vi "SetGroupProperty.vi"(7 "LabVIEW Web Service Request":refnum<class "Web Request.lvclass">) -> ()   [LabVIEW 2018]
uses:
  <vilib>/wsapi/Web Request.lvclass
  subvis/Group Properties.ctl
  CAEN globals.vi
panel:
  in  "error in (no error)":errorcluster
  # "Use the Web Service Request input terminal to call the VIs on the Web Services palette. Do not remove it from the connector pane unless you don't need access to the palette."
  # "Each additional control wired to the connector pane will be available as an input in the URL. To include an indicator in terminal-mode output (the default setting), it must also be wired to the connector pane."
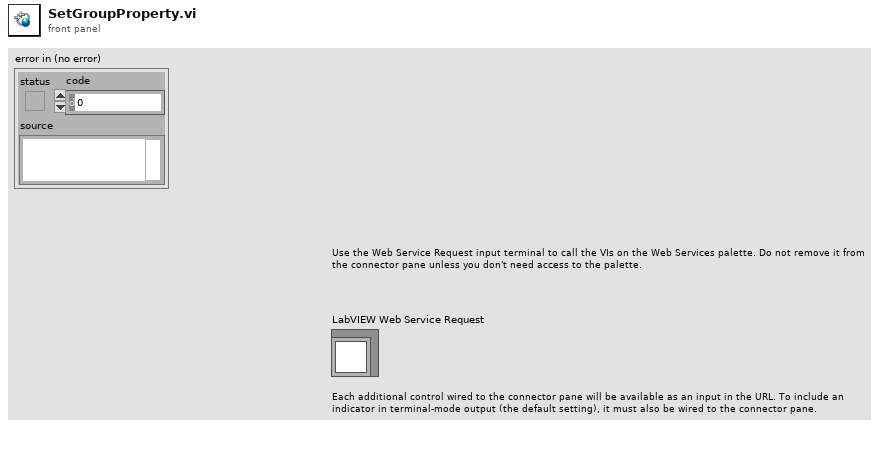
[diagram p1: front panel]
types:
  T1 = typedef "Group Properties.ctl" = enum16{"Enable", "Vset", "Imax", "Vswmax", "Trip Time"}
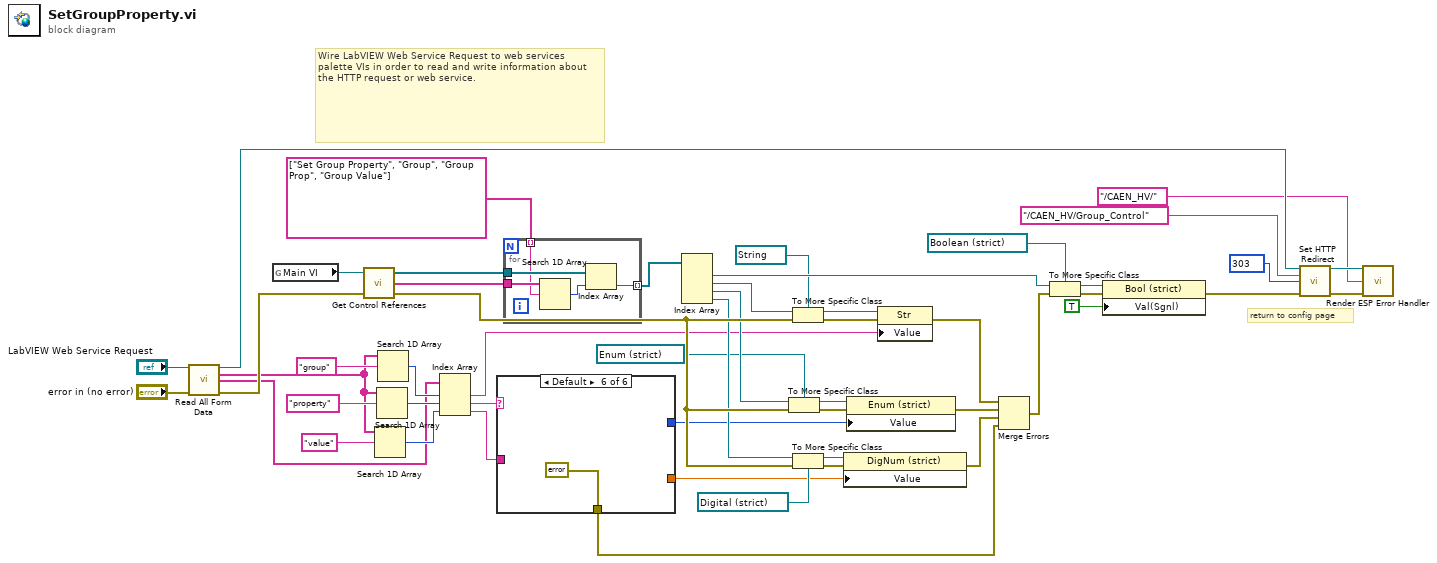
[diagram p0: block diagram]
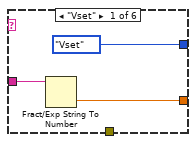
[diagram p2: hidden frame]
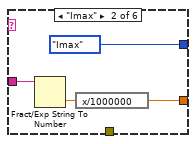
[diagram p3: hidden frame]
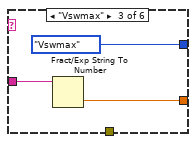
[diagram p4: hidden frame]
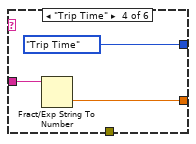
[diagram p5: hidden frame]
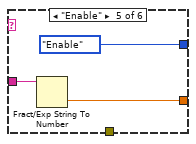
[diagram p6: hidden frame]
diagram:
  w46 = 303 items=["100"=100, "101"=101, "200"=200, "201"=201, "202"=202, "203"=203, "204"=204, "205"=205, "206"=206, "300"=300, "301"=301, "302"=302, "303"=303, "304"=304, "305"=305, "306"=306, "307"=307, "400"=400, "401"=401, "402"=402, "403"=403, "404"=404, "405"=405, "406"=406, "407"=407, "408"=408, "409"=409, "410"=410, "411"=411, "412"=412, "413"=413, "414"=414, "415"=415, "416"=416, "417"=417, "500"=500, "501"=501, "502"=502, "503"=503, "504"=504, "505"=505] ("response code (307)")
  # "return to config page"
  # "Wire LabVIEW Web Service Request to web services palette VIs in order to read and write information about the HTTP request or web service."
  n1 = call <vilib>:"Read All Form Data.vi"("LabVIEW Web Service Request"="LabVIEW Web Service Request", "error in (no error)"="error in (no error)") -> ("LabVIEW Web Service Request out"=w22:refnum<class "Web Request.lvclass">, "Key"=w14:string[], "Value"=w12:string[], "error out"=w23:errorcluster)  [unwired: 9 in, 1 out]
  n2 = global read "CAEN globals.vi" "Main VI"() -> (w51:refnum<vi>)
  n3 = call "Get Control References.vi"("error in"=w23, "This vi"=w51) -> ("error out"=w25:errorcluster, "Control Names"=w50:string[], "Controls[]"=w49:refnum<vi>[])  [unwired: 1 in]
  n4 = Search 1D Array(1D array=w14, element="value") -> (index of element=w13:i32)  [unwired: 1 in]
  n5 = Search 1D Array(1D array=w14, element="property") -> (index of element=w41:i32)  [unwired: 1 in]
  n6 = Search 1D Array(1D array=w14, element="group") -> (index of element=w42:i32)  [unwired: 1 in]
  n7 = Index Array(array=w12, index #1=w42, index #2=w41, index #3=w13) -> (element #1=w8:string, element #2=w5:string, element #3=w3:string)
  n8 = case shown="Default" w5 {
    tunnel: [Group_Properties."Vset" ("Value") Group_Properties."Imax" ("Value") Group_Properties."Vswmax" ("Value") Group_Properties."Trip Time" ("Value") Group_Properties."Enable" ("Value") _] -> w4
    tunnel: w3 -> [w53 w56 w60 w63 w66 _]
    tunnel: [w52 w55 w59 w62 w65 _] -> w2
    tunnel: [_ _ _ _ _ errorcluster {"status"=TRUE, "code"=0, "source"="Unrecognised group property"} ("error out")] -> w1
    frame "Vset" {
      n9 = Fract/Exp String To Number(string=w53) -> (number=w52:dbl)  [unwired: 3 in, 1 out]
    }
    frame "Imax" {
      n10 = Fract/Exp String To Number(string=w56) -> (number=w57:dbl)  [unwired: 3 in, 1 out]
      n11 = expression code="x/1000000"(w57) -> (w55:dbl)
    }
    frame "Vswmax" {
      n12 = Fract/Exp String To Number(string=w60) -> (number=w59:dbl)  [unwired: 3 in, 1 out]
    }
    frame "Trip Time" {
      n13 = Fract/Exp String To Number(string=w63) -> (number=w62:dbl)  [unwired: 3 in, 1 out]
    }
    frame "Enable" {
      n14 = Fract/Exp String To Number(string=w66) -> (number=w65:dbl)  [unwired: 3 in, 1 out]
    }
    frame Default {
    }
  }
  n15 = for {
    tunnel: w50 -> [w73]
    tunnel: w49 -> [w72]
    tunnel: [w70] -> w20 mode=indexing
    tunnel: string[] ["Set Group Property", "Group", "Group Prop", "Group Value"] ("Control Names") -> [w69] mode=indexing
    n16 = Search 1D Array(1D array=w73, element=w69) -> (index of element=w71:i32)  [unwired: 1 in]
    n17 = Index Array(array=w72, index=w71) -> (element=w70:refnum<vi>)
  }
  n18 = Index Array(array=w20) -> (element #1=w19:refnum<vi>, element #2=w18:refnum<vi>, element #3=w17:refnum<vi>, element #4=w16:refnum<vi>)  [unwired: 4 in]
  n19 = To More Specific Class(target class=refnum<vi> refnum ("Group Prop"), reference=w17, error in=w25) -> (specific class reference=w38:refnum<vi>, error out=w37:errorcluster)
  n20 = To More Specific Class(target class=refnum<vi> refnum ("element"), reference=w18, error in=w25) -> (specific class reference=w47:refnum<vi>, error out=w48:errorcluster)
  n21 = To More Specific Class(target class=refnum<vi> refnum ("Numeric Control"), reference=w16, error in=w25) -> (specific class reference=w35:refnum<vi>, error out=w36:errorcluster)
  n22 = property class="DigNum (strict)"(reference=w35, error in=w36, "Value"=w2) -> (error out=w29:errorcluster)  [unwired: 1 out]
  n23 = property class="Enum (strict)"(reference=w38, error in=w37, "Value"=w4) -> (error out=w28:errorcluster)  [unwired: 1 out]
  n24 = property class="Str"(reference=w47, error in=w48, "Value"=w8) -> (error out=w27:errorcluster)  [unwired: 1 out]
  n25 = Merge Errors(w27, w28, w29, w1) -> (w26:errorcluster)
  n26 = To More Specific Class(target class=refnum<vi> refnum ("replace all? (F)"), reference=w19, error in=w26) -> (specific class reference=w33:refnum<vi>, error out=w32:errorcluster)
  n27 = property class="Bool (strict)"(reference=w33, error in=w32, "Val(Sgnl)"=TRUE ("Value (Signaling)")) -> (error out=w30:errorcluster)  [unwired: 1 out]
  n28 = call <vilib>:"Set HTTP Redirect.vi"("LabVIEW Web Service Request"=w22, "redirect URL"="/CAEN_HV/Group_Control", "response code (307)"=w46, "error in (no error)"=w30) -> ("LabVIEW Web Service Request out"=w44:refnum<class "Web Request.lvclass">, "error out"=w45:errorcluster)  [unwired: 10 in]
  n29 = call "Render ESP Error Handler.vi"("LabVIEW Web Service Request"=w44, "Link"="/CAEN_HV/" ("redirect URL"), "error in (no error)"=w45) -> ()  [unwired: 11 in, 2 out]
